vi "WPI_CameraBasisString.vi"(11 "Input Mode":T1) -> (2 "Basis":string, 3 "length":i32)   [LabVIEW 2017]
panel:
  out "Array 3":i32[](array[numeric])
  out "Array 2":i32[](array[numeric])
  out "Array":string[](array[string])
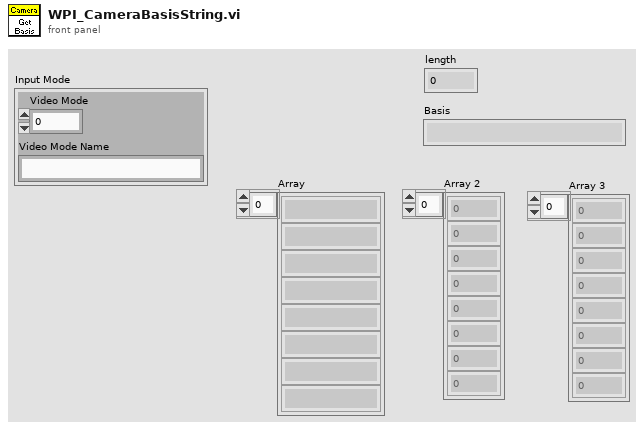
[diagram p1: front panel]
types:
  T1 = cluster{"Video Mode":u32, "Video Mode Name":string}
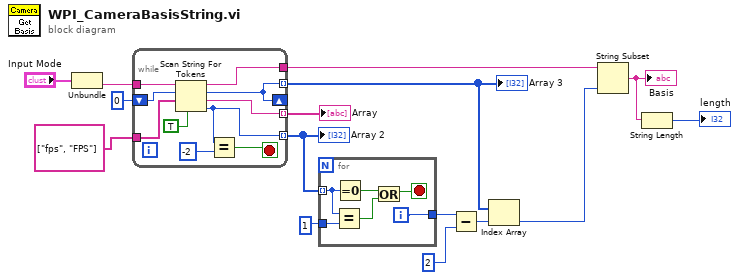
[diagram p0: block diagram]
diagram:
  n1 = Unbundle("Input Mode") -> ("Video Mode Name"=w1:string)  [unwired: 1 out]
  n2 = while {
    tunnel: w1 -> [w25]
    shift-right: [w17] -> _
    shift-left: 0 ("offset past token") -> [w24]
    tunnel: [w22] -> w14 mode=indexing
    tunnel: string[] ["fps", "FPS"] -> [w19]
    tunnel: [w18] -> w12 mode=indexing
    tunnel: [w17] -> w8 mode=indexing
    tunnel: [w16] -> w7
    stop <- w20 stop-if-true
    n3 = Scan String For Tokens(4:TRUE ("use cached delim/oper data? (F)"), 7:w19, 8:w24, 9:w25) -> (0:w18:i32, 1:w22:string, 2:w17:i32, 3:w16:string)  [unwired: 2 in]
    n4 = Equal?(x=w18, y=-2) -> (x = y?=w20:bool)
  }
  "Array" <- w14
  "Array 2" <- w12
  "Array 3" <- w8
  n5 = for {
    tunnel: w12 -> [w28] mode=indexing
    tunnel: [w30] -> w10
    tunnel: 1 ("y") -> [w26]
    i -> [w30]
    stop <- w29 stop-if-true
    n6 = Equal?(x=w28, y=w26) -> (x = y?=w27:bool)
    n7 = Equal To 0?(x=w28) -> (x = 0?=w31:bool)
    n8 = Or(x=w31, y=w27) -> (x .or. y?=w29:bool)
  }
  n9 = Subtract(x=w10, y=2) -> (x-y=w9:i32)
  n10 = Index Array(array=w8, index=w9) -> (element=w6:i32)
  n11 = String Subset(string=w7, length (rest)=w6) -> (substring=w4:string)  [unwired: 1 in]
  "Basis" <- w4
  n12 = String Length(string=w4) -> (length=→"length":i32)
